vi "LJM_eStreamRead2D.vi"(0 "Handle In":i32, 5 "ScansPerRead":i32, 7 "NumAddresses":i32, 11 "error in":errorcluster) -> (4 "Handle Out":i32, 6 "aData Out":dbl[][](array[numeric]), 13 "DeviceScanBacklog":i32, 14 "LJMScanBacklog":i32, 15 "error out":errorcluster)   [LabVIEW 2020]
uses:
  Library/Frameworks/LabJackM.framework
panel:
  # "Uses \"Reentrant\" for the DLL call."
  # "These 2 are not actually parameters of the\neStreamRead function, but we pass them\nto this VI so it can initialize the array.  Pass\nin the same values passed to eStreamStart."
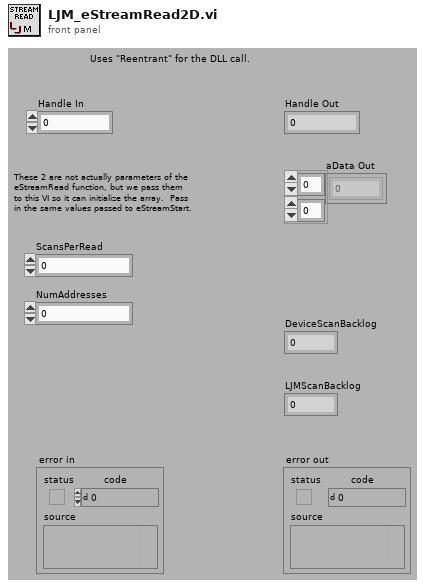
[diagram p1: front panel]
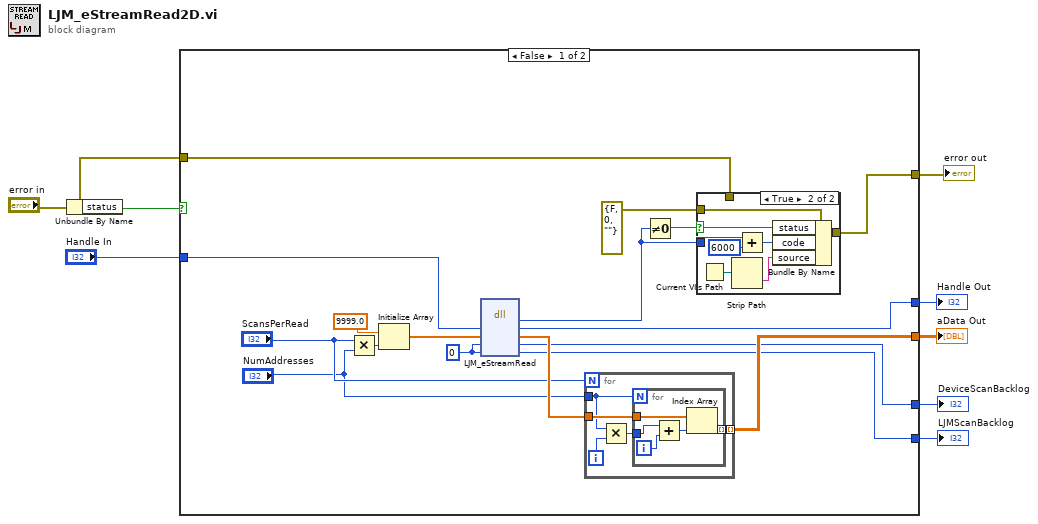
[diagram p0: block diagram]
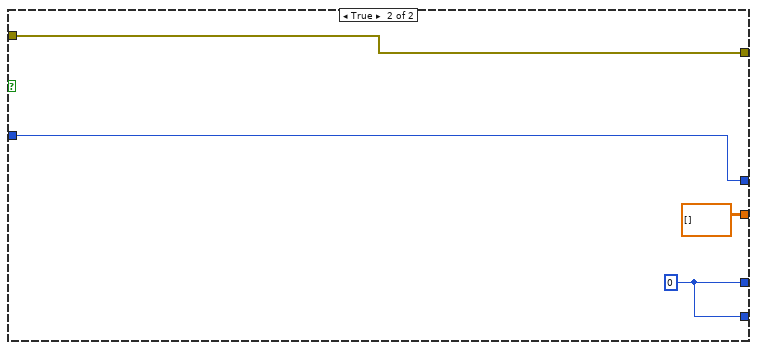
[diagram p3: hidden frame]
diagram:
  n1 = Unbundle By Name("error in") -> ("status"=w8:bool)
  n2 = case shown="False" w8 {
    tunnel: "error in" -> [w21 w48]
    tunnel: [w22 w48] -> w7
    tunnel: [w20 w47] -> w6
    tunnel: "Handle In" -> [w19 w47]
    tunnel: [w13 dbl[][] []] -> w4
    tunnel: [w10 w46] -> w3
    tunnel: [w9 w46] -> w2
    frame False {
      w18 = 0 ("NumSkippedScans")
      n3 = Multiply(x="ScansPerRead", y="NumAddresses") -> (x*y=w15:i32)
      n4 = Initialize Array(9999.0 ("element"), w15) -> (w17:dbl[])
      n5 = dll-call lib="Library/Frameworks/LabJackM.framework" fn="LJM_eStreamRead"("Handle"=w19, "aData"=w17, "DeviceScanBacklog"=w18, "LJMScanBacklog"=w18) -> ("return type"=w25:i32, "Handle"=w20:i32, "aData"=w14:dbl[], "DeviceScanBacklog"=w10:i32, "LJMScanBacklog"=w9:i32)  [unwired: 3 in, 2 out]
      n6 = for {
        N: "ScansPerRead" -> [_]
        tunnel: "NumAddresses" -> [w28]
        tunnel: w14 -> [w30]
        tunnel: [w26] -> w13 mode=indexing
        i -> [w29]
        n7 = Multiply(x=w28, y=w29) -> (x*y=w27:i32)
        n8 = for {
          N: w28 -> [_]
          tunnel: w30 -> [w35]
          tunnel: w27 -> [w32]
          tunnel: [w31] -> w26 mode=indexing
          i -> [w33]
          n9 = Add(x=w32, y=w33) -> (x+y=w34:i32)
          n10 = Index Array(array=w35, index=w34) -> (element=w31:dbl)
        }
      }
      n11 = Not Equal To 0?(x=w25) -> (x != 0?=w24:bool)
      n12 = case shown="True" w24 {
        selector: w24 -> [_ w43]
        tunnel: [w36 w44] -> w22
        tunnel: errorcluster {"status"=FALSE, "code"=0, "source"=""} ("error IO") -> [_ w42]
        tunnel: w25 -> [_ w38]
        tunnel: w21 -> [w36 _]
        frame False {
        }
        frame True {
          n13 = Current VI's Path() -> (path=w40:path)
          n14 = Strip Path(path=w40) -> (name=w41:string)  [unwired: 1 out]
          n15 = Add(x=w38, y=6000) -> (x+y=w39:i32)
          n16 = Bundle By Name(cluster=w42, "status"=w43, "code"=w39, "source"=w41) -> (w44:errorcluster)
        }
      }
    }
    frame True {
      w46 = 0 ("NumSkippedScans")
    }
  }
  "error out" <- w7
  "Handle Out" <- w6
  "aData Out" <- w4
  "DeviceScanBacklog" <- w3
  "LJMScanBacklog" <- w2
